vi "Set ITEMP Voltage.vi"(7 "Position in":u32, 8 "Error in":errorcluster caption="Error in (no error)", 10 "Voltage":dbl, 11 "Calibration in":refnum<class "Calibration.lvclass">) -> (0 "Error out":errorcluster, 2 "Channel":string, 3 "Power Supply":refnum<class "Power Supply.lvclass">)   [LabVIEW 2015, in "Calibration.lvclass"]
uses:
  Calibration.lvclass
  Classes/Instruments/Power Supply/Class/Power Supply.lvclass
  CBTF Applications/Driver Board Testing/Main/Application/Application/Class/typedefs/Instrument Selector -- Enum.ctl
  CBTF Applications/Driver Board Testing/Main/Application/Application/Class/Driver Board Test.lvclass
  Test Class/Test Class.lvclass
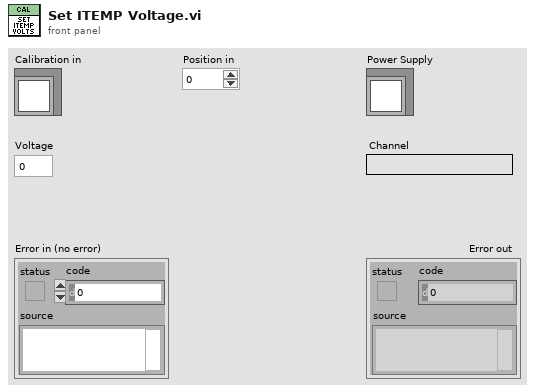
[diagram p1: front panel]
types:
  T1 = typedef "Driver Board Test.lvlib/Driver Board Test.lvclass/Instrument Selector -- Enum.ctl" = enum16{"ACPS1", "ACPS2", "DCPS1", "DCPS2", "DCPS3", "DCLoad1", "DCLoad2", "DPM1", "DPM2", "Switch1", "PXI1Slot2", "PXI1Slot3", "cDAQ1Mod5", "cDAQ1Mod6", "cDAQ1Mod7", "cDAQ1Mod8", "cDAQ1Mod1", "cDAQ1Mod2", "cDAQ1Mod3", "cDAQ1Mod4", "cDAQ2Mod1", "cDAQ2Mod2", "cDAQ2Mod3", "cDAQ2Mod4"}
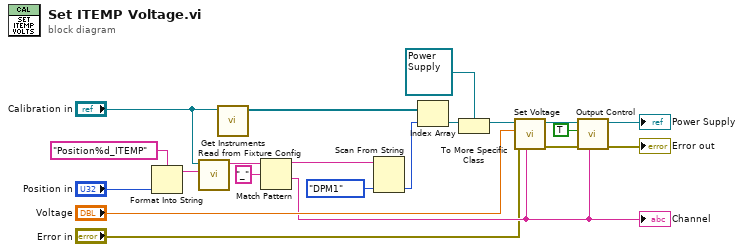
[diagram p0: block diagram]
diagram:
  n1 = Format Into String(format string="Position%d_ITEMP" ("String"), "Position in") -> (resulting string=w4:string)  [unwired: 2 in, 1 out]
  n2 = call-dynamic "Read from Fixture Config.vi"("Key"=w4, "Test Class in"="Calibration in") -> ("Instrument Info"=w1:string)  [unwired: 8 in, 1 out]
  n3 = call "Get Instruments.vi"("Test Class in"="Calibration in") -> ("Instruments"=w2:refnum<class "Instrument.lvclass">[])  [unwired: 9 in, 1 out]
  n4 = Match Pattern(string=w1, regular expression="_") -> (before substring=w19:string, after substring=w10:string)  [unwired: 1 in, 2 out]
  "Channel" <- w10
  n5 = Scan From String(input string=w19, default 1=Instrument_Selector_--_Enum."DPM1" ("Instrument")) -> (output 1=w18:T1)  [unwired: 3 in, 3 out]
  n6 = Index Array(array=w2, index=w18) -> (element=w17:refnum<class "Instrument.lvclass">)
  n7 = To More Specific Class(target class=refnum<class "Power Supply.lvclass"> refnum ("Power Supply.lvlib:Power Supply.lvclass"), reference=w17) -> (specific class reference=w15:refnum<class "Power Supply.lvclass">)  [unwired: 1 in, 1 out]
  n8 = call-dynamic "Set Voltage.vi"("Channel (\"1\")"=w10, "error in (no error)"="Error in", "Voltage (0.0 V)"="Voltage", "Acrobat Template in"=w15) -> ("error out"=w7:errorcluster, "Acrobat Template out"=w11:refnum<class "Power Supply.lvclass">)  [unwired: 6 in]
  n9 = call-dynamic "Output Control.vi"("Channel (\"1\")"=w10, "error in (no error)"=w7, "Enabled"=TRUE, "Acrobat Template in"=w11) -> ("error out"=→"Error out":errorcluster, "Acrobat Template out"=→"Power Supply":refnum<class "Power Supply.lvclass">)  [unwired: 6 in]
